vi "Write Filter Wheel Info.vi"(8 "error in (no error)":errorcluster, 10 "Filter Wheel Info":T1={"Num Wheels"=0, "Filters"=[], "Invalid Combinations"=[], "Addr"="", "Name"="", "Simulate"=FALSE, "Homing Parameters"={"Direction (F: CW)"=TRUE, "Speed"=150, "Accel"=400, "Min Distance"=2700, "Short Leg"=0, "Error Cnts"=0}, "Default Speed"=1000} {"Default Speed" min=20 max=4000 step=10}, 11 "Filter Wheel in":refnum<class "Filter Wheel.lvclass">) -> (0 "error out":errorcluster, 3 "Filter Wheel out":refnum<class "Filter Wheel.lvclass">)   [LabVIEW 2024, in "Filter Wheel.lvclass"]
uses:
  Filter Wheel.lvclass
  Filter Wheel configuration.ctl
  Filter Wheel Details.ctl
  Filter Wheel Arduino Control/Filter Wheel Arduino Homing cluster.ctl
  Filter Wheel.lvclass/Filter Wheel.ctl
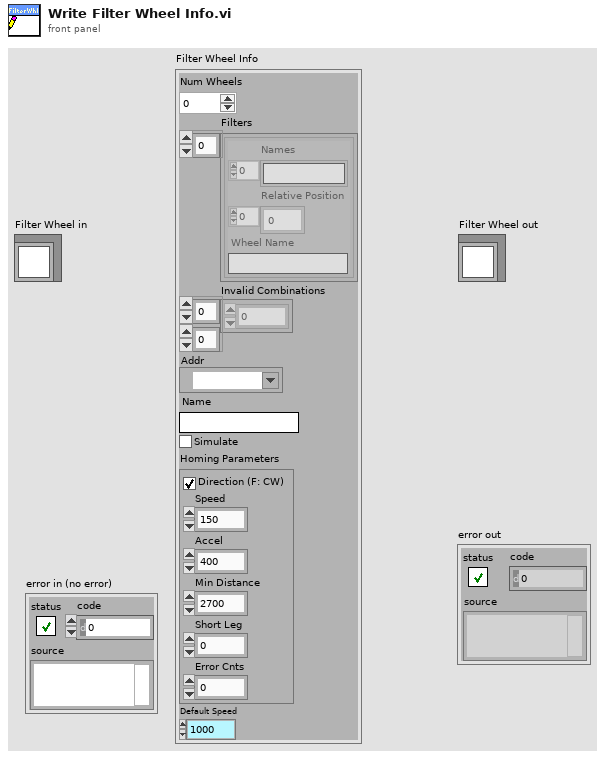
[diagram p1: front panel]
types:
  T1 = typedef "Filter Wheel.lvclass/Filter Wheel configuration.ctl" = cluster{"Num Wheels":i32, "Filters":T2[], "Invalid Combinations":i32[][], "Addr":refnum<visa-resource-name>, "Name":string, "Simulate":bool, "Homing Parameters":T3, "Default Speed":u16}
  T2 = typedef "Filter Wheel.lvclass/Filter Wheel Details.ctl" = cluster{"Names":string[], "Relative Position":i32[], "Wheel Name":string}
  T3 = typedef "Filter Wheel Arduino Homing cluster.ctl" = cluster{"Direction (F: CW)":bool, "Speed":i32, "Accel":i32, "Min Distance":i32, "Short Leg":i32, "Error Cnts":i32}
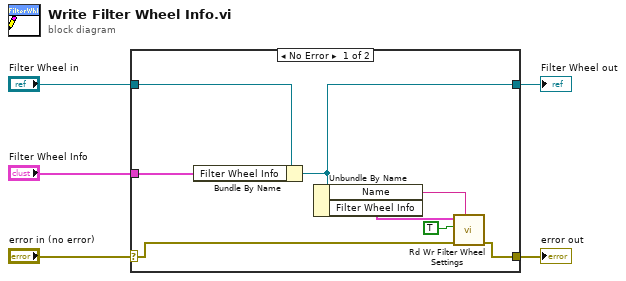
[diagram p0: block diagram]
diagram:
  n1 = case shown="No Error" "error in (no error)" {
    selector: "error in (no error)" -> [w9 w14]
    tunnel: [w8 w14] -> w4
    tunnel: [w11 w15] -> w2
    tunnel: "Filter Wheel in" -> [w13 w15]
    tunnel: "Filter Wheel Info" -> [w12 _]
    frame No Error {
      n2 = Bundle By Name(cluster=w13, "Filter Wheel Info"=w12) -> (w11:refnum<class "Filter Wheel.lvclass">)
      n3 = Unbundle By Name(w11) -> ("Name"=w6:string, "Filter Wheel Info"=w10:T1)
      n4 = call "Rd Wr Filter Wheel Settings.vi"("Wheel Name"=w6, "error in (no error)"=w9, "Write? (F:Read)"=TRUE, "Filter Wheel Settings"=w10) -> ("error out"=w8:errorcluster)  [unwired: 6 in, 1 out]
    }
    frame Error {
    }
  }
  "error out" <- w4
  "Filter Wheel out" <- w2
